vi "CODcr启动器.vi"(11 "控制命令":enum16{"水样测试", "平行样测试", "加标回收", "停止"}(ring)) -> ()   [LabVIEW 2016, in "质控单元V1.lvlib"]
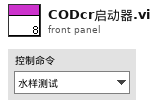
[diagram p1: front panel]
types:
  T1 = cluster{"站号":u16, "量程切换":enum32{"H", "L", "AUTO"}, "控制命令":enum16{"启动测量", "标样核查", "零点核查", "跨度核查", "空白测试", "平行样测试", "加标回收", "空白校准", "标样校准", "初始化（清洗）", "停止测试", "仪器重启", "校时", "模式设置", "测量间隔设置"}, "模式设置":enum16{"待机", "连续模式", "周期模式", "定点模式", "受控模式", "手动模式"}, "测量间隔":u16}
  T2 = enum16{"启动测量", "标样核查", "零点核查", "跨度核查", "空白测试", "平行样测试", "加标回收", "空白校准", "标样校准", "初始化（清洗）", "停止测试", "仪器重启", "校时", "模式设置", "测量间隔设置"}
  T3 = cluster{"命令":string, "测量模式":enum16{"水样测量", "标样核查", "零点核查", "跨度核查", "空白测试", "加标回收", "平行样", "校零", "校标"}, "CODMn量程切换":enum32{"H", "L", "AUTO"}}
  T4 = enum16{"水样测量", "标样核查", "零点核查", "跨度核查", "空白测试", "加标回收", "平行样", "校零", "校标"}
  T5 = cluster{"水样测试量程模式":enum16{"H", "L", "AUTO"}, "空白核查量程模式":enum16{"H", "L", "AUTO"}, "跨度核查量程模式":enum16{"H", "L", "AUTO"}, "加标回收量程模式":enum16{"H", "L", "AUTO"}}
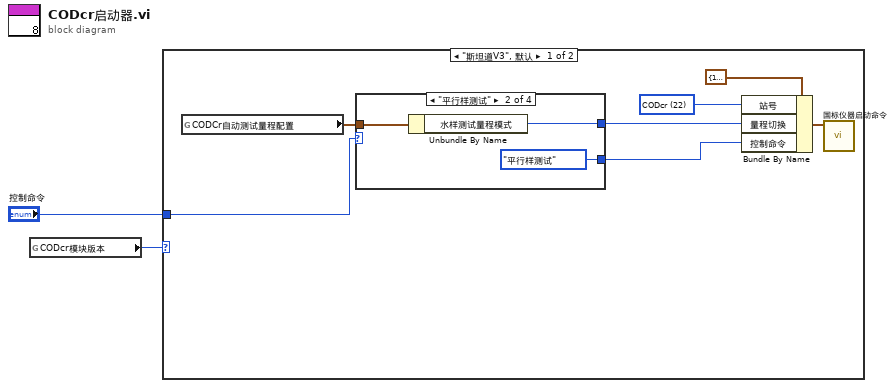
[diagram p0: block diagram]
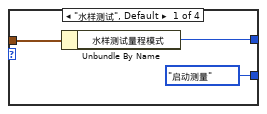
[diagram p2: hidden frame]
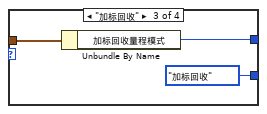
[diagram p3: hidden frame]
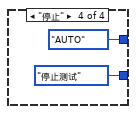
[diagram p4: hidden frame]
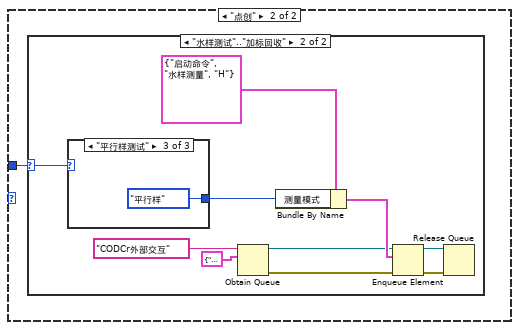
[diagram p5: hidden frame]
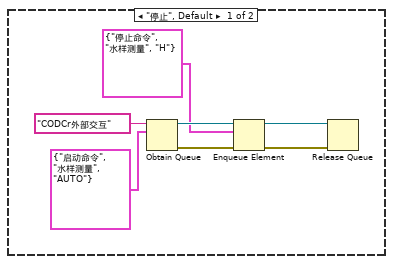
[diagram p6: hidden frame]
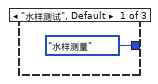
[diagram p7: hidden frame]
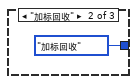
[diagram p8: hidden frame]
diagram:
  n1 = global read "系统交互.vi" "CODcr模块版本"() -> (w2:enum16{"斯坦道V3", "点创"})
  n2 = case shown="\"斯坦道V3\", 默认" w2 {
    tunnel: "控制命令" -> [w3 w21]
    frame "斯坦道V3", Default {
      w4 = u16 22 items=["总磷"=1, "总氮"=2, "氨氮"=3, "CODMn"=21, "CODcr"=22] ("站号")
      n3 = global read "系统交互.vi" "CODCr自动测试量程配置"() -> (w7:T5)
      n4 = case shown="\"平行样测试\"" w3 {
        tunnel: [T2."启动测量" T2."平行样测试" T2."加标回收" T2."停止测试"] -> w9
        tunnel: w7 -> [w11 w14 w17 _]
        tunnel: [w10 w13 w16 enum16{"H", "L", "AUTO"}."AUTO" ("加标回收量程模式")] -> w8
        frame "水样测试", Default {
          n5 = Unbundle By Name(w11) -> ("水样测试量程模式"=w10:enum16{"H", "L", "AUTO"})
        }
        frame "平行样测试" {
          n6 = Unbundle By Name(w14) -> ("水样测试量程模式"=w13:enum16{"H", "L", "AUTO"})
        }
        frame "加标回收" {
          n7 = Unbundle By Name(w17) -> ("加标回收量程模式"=w16:enum16{"H", "L", "AUTO"})
        }
        frame "停止" {
        }
      }
      n8 = Bundle By Name(cluster=T1 {"站号"=1, "量程切换"=enum."AUTO", "控制命令"=enum."启动测量", "模式设置"=enum."待机", "测量间隔"=0} ("参数"), "站号"=w4, "量程切换"=w8, "控制命令"=w9) -> (w5:T1)
      n9 = call "国标仪器启动命令.vi"("参数"=w5) -> ()  [unwired: 10 in, 1 out]
    }
    frame "点创" {
      n10 = case shown="\"水样测试\"..\"加标回收\"" w21 {
        selector: w21 -> [_ w38]
        frame "停止", Default {
          n11 = Obtain Queue(name (unnamed)="CODCr外部交互" ("名称（未命名）"), element data type=T3 {"命令"="启动命令", "测量模式"=enum."水样测量", "CODMn量程切换"=enum."AUTO"} ("元素")) -> (queue out=w24:refnum<queue>, error out=w23:errorcluster)  [unwired: 3 in, 1 out]
          n12 = Enqueue Element(queue=w24, element=T3 {"命令"="停止命令", "测量模式"=enum."水样测量", "CODMn量程切换"=enum."H"} ("元素"), error in (no error)=w23) -> (queue out=w26:refnum<queue>, error out=w25:errorcluster)  [unwired: 1 in, 1 out]
          n13 = Release Queue(queue=w26, error in (no error)=w25) -> ()  [unwired: 1 in, 3 out]
        }
        frame "水样测试".."加标回收" {
          n14 = case shown="\"平行样测试\"" w38 {
            tunnel: [T4."水样测量" ("测量模式") T4."加标回收" ("测量模式") T4."平行样" ("测量模式")] -> w29
            frame "水样测试", Default {
            }
            frame "加标回收" {
            }
            frame "平行样测试" {
            }
          }
          n15 = Obtain Queue(name (unnamed)="CODCr外部交互" ("名称（未命名）"), element data type=T3 {"命令"="启动命令", "测量模式"=enum."水样测量", "CODMn量程切换"=enum."AUTO"} ("元素")) -> (queue out=w31:refnum<queue>, error out=w30:errorcluster)  [unwired: 3 in, 1 out]
          n16 = Bundle By Name(cluster=T3 {"命令"="启动命令", "测量模式"=enum."水样测量", "CODMn量程切换"=enum."H"} ("元素"), "测量模式"=w29) -> (w32:T3)
          n17 = Enqueue Element(queue=w31, element=w32, error in (no error)=w30) -> (queue out=w35:refnum<queue>, error out=w34:errorcluster)  [unwired: 1 in, 1 out]
          n18 = Release Queue(queue=w35, error in (no error)=w34) -> ()  [unwired: 1 in, 3 out]
        }
      }
    }
  }
